vi "Truncate_Cluster.vi"() -> ()   [LabVIEW 2015]
uses:
  System Monitor Cluster.ctl
panel:
  in  "System Monitor Variables":T1={"Time"=[], "LI1CH1"=[], "LI1CH2"=[], "LI2CH1"=[], "LI2CH2"=[], "LI3CH1"=[], "LI3CH2"=[], "Field"=[], "Temperature"=[], "Temperature 2"=[], "Temperatrue 3"=[], "Nitrogen Level"=[], "Helium Level"=[], "Heater LS370"=[], "Sorb Heater"=[], "Still Heater"=[], "Capacity"=[], "Loss"=[], "Magnet Temperature"=[], "Lambda Pressure"=[], "Lambda Needle Valve"=[], "LS370-CH1-T"=[], "LS370-CH2-T"=[], "LS370-CH3 -T"=[], "LS370-CH1-R"=[], "LS370-CH2-R"=[], "LS370-CH3-R"=[], "LS372-CH1-T"=[], "LS372-CH2-T"=[], "LS372-CH3 -T"=[], "LS372-CH1-R"=[], "LS372-CH2-R"=[], "LS372-CH3-R"=[], "Nada"=[nan], "Keithley Res"=[], "Keithley Current"=[], "VTI Heater"=[], "VTI Needle Valve"=[], "VTI Needle Valve 2"=[]}
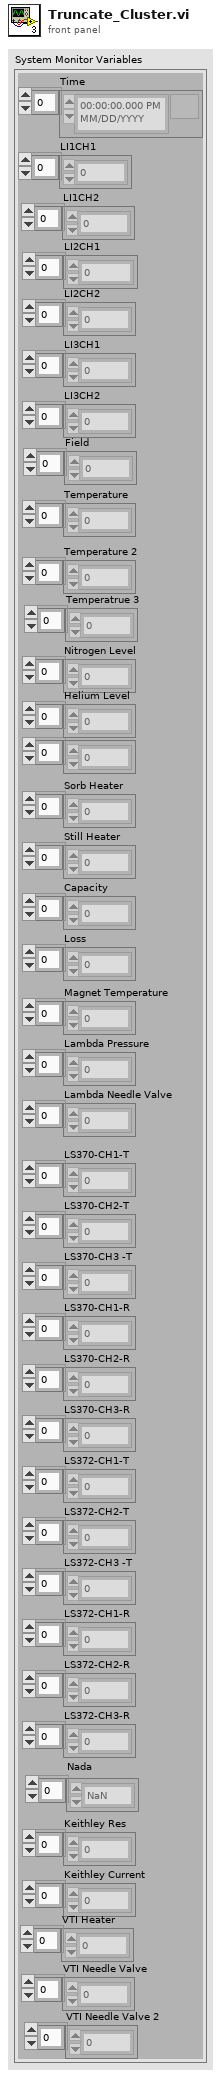
[diagram p1: front panel]
types:
  T1 = typedef "System Monitor Cluster.ctl" = cluster{"Time":timestamp[], "LI1CH1":dbl[], "LI1CH2":dbl[], "LI2CH1":dbl[], "LI2CH2":dbl[], "LI3CH1":dbl[], "LI3CH2":dbl[], "Field":dbl[], "Temperature":dbl[], "Temperature 2":dbl[], "Temperatrue 3":dbl[], "Nitrogen Level":dbl[], "Helium Level":dbl[], "Heater LS370":dbl[], "Sorb Heater":dbl[], "Still Heater":dbl[], "Capacity":dbl[], "Loss":dbl[], "Magnet Temperature":dbl[], "Lambda Pressure":dbl[], "Lambda Needle Valve":dbl[], "LS370-CH1-T":dbl[], "LS370-CH2-T":dbl[], "LS370-CH3 -T":dbl[], "LS370-CH1-R":dbl[], "LS370-CH2-R":dbl[], "LS370-CH3-R":dbl[], "LS372-CH1-T":dbl[], "LS372-CH2-T":dbl[], "LS372-CH3 -T":dbl[], "LS372-CH1-R":dbl[], "LS372-CH2-R":dbl[], "LS372-CH3-R":dbl[], "Nada":dbl[], "Keithley Res":dbl[], "Keithley Current":dbl[], "VTI Heater":dbl[], "VTI Needle Valve":dbl[], "VTI Needle Valve 2":dbl[]}
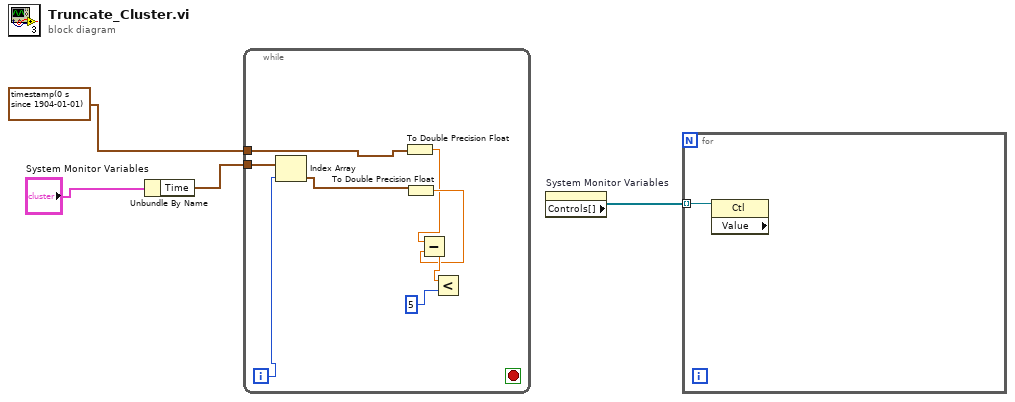
[diagram p0: block diagram]
diagram:
  n1 = Unbundle By Name("System Monitor Variables") -> ("Time"=w2:timestamp[])
  n2 = while {
    tunnel: w2 -> [w7]
    tunnel: timestamp(0 s since 1904-01-01) -> [w6]
    i -> [w8]
    stop <- _ stop-if-true
    n3 = Index Array(array=w7, index=w8) -> (element=w5:timestamp)
    n4 = To Double Precision Float(number=w6) -> (double precision float=w9:dbl)
    n5 = To Double Precision Float(number=w5) -> (double precision float=w10:dbl)
    n6 = Subtract(x=w9, y=w10) -> (x-y=w11:dbl)
    n7 = Less?(x=w11, y=5) -> ()  [unwired: 1 out]
  }
  n8 = property on="System Monitor Variables" class="Clust (strict)"() -> ("Controls[]"=w4:refnum<vi>[])  [unwired: 2 in, 2 out]
  n9 = for {
    tunnel: w4 -> [w13] mode=indexing
    n10 = property class="Ctl" props=["Value"](reference=w13) -> ()  [unwired: 1 in, 3 out]
  }
